vi "CreateFoldersRecursively.vi"(8 "error in (no error)":errorcluster caption="错误输入（无错误）", 9 "permissions":i16=493 caption="权限" format="%.0b", 10 "maximum path length":i32=252 caption="路径长度上限", 11 "directory":path caption="目录") -> (0 "error out":errorcluster caption="错误输出", 2 "directories created":path[](array[path]) caption="创建的目录", 3 "directory copy":path caption="目录副本")   [LabVIEW 2019, in "Logger.lvclass"]
uses:
  <userlib>/Logger/Logger.lvclass
panel:
  in  "Long Path Message":string="由于操作系统限制，该完整路径包含过多字符，LabVIEW将无法创建该文件夹。" caption="长路径信息"
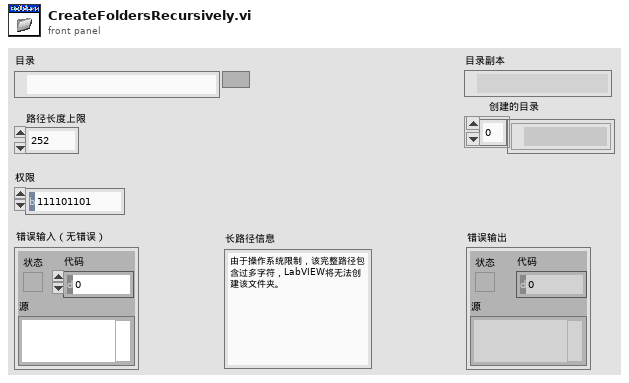
[diagram p1: front panel]
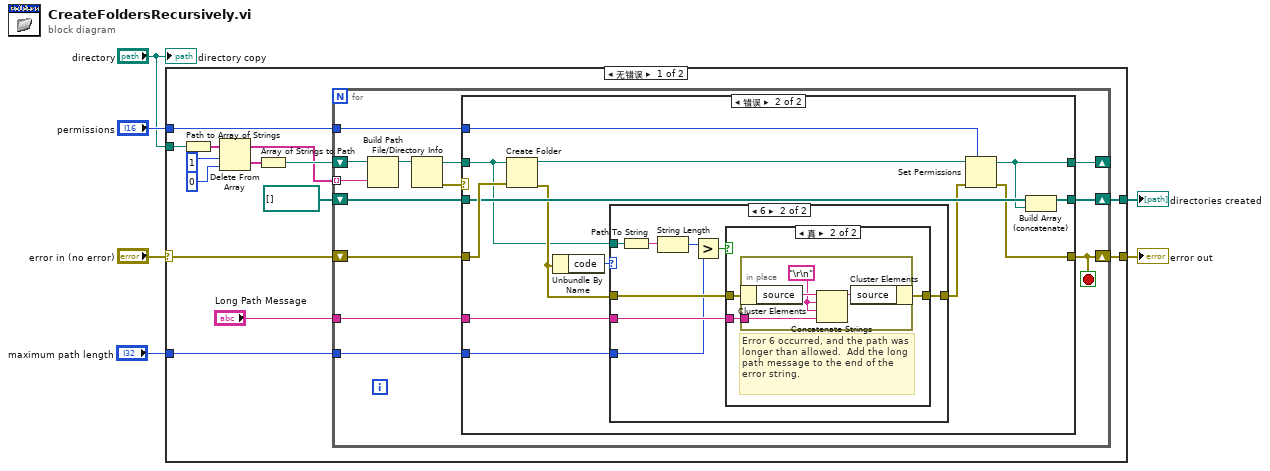
[diagram p0: block diagram]
diagram:
  n1 = case shown="无错误" "error in (no error)" {
    selector: "error in (no error)" -> [w9 w67]
    tunnel: [w20 w67] -> w6
    tunnel: "permissions" -> [w19 _]
    tunnel: [w15 _] -> w4
    tunnel: "directory" -> [w12 _]
    tunnel: "maximum path length" -> [w7 _]
    frame No Error {
      n2 = Path to Array of Strings(0:w12) -> (2:w18:string[])  [unwired: 1 out]
      n3 = Delete From Array(array=w18, length=1, index=0) -> (deleted portion=w13:string[], array with subset deleted=w10:string[])
      n4 = Array of Strings to Path(0:w13) -> (2:w17:path)  [unwired: 1 out]
      n5 = for {
        shift-right: [w29] -> _
        shift-left: w17 -> [w33]
        tunnel: w10 -> [w32] mode=indexing
        shift-right: [w23] -> w20
        shift-left: w9 -> [w28]
        tunnel: w19 -> [w27]
        shift-right: [w25] -> w15
        shift-left: path[] [] ("Array Constant") -> [w26]
        tunnel: "Long Path Message" -> [w22]
        tunnel: w7 -> [w21]
        stop <- w23 stop-if-true
        n6 = Build Path(base path=w33, name or relative path=w32) -> (appended path=w31:path)
        n7 = File/Directory Info(path=w31) -> (path out=w30:path, error out=w24:errorcluster)  [unwired: 1 in, 5 out]
        n8 = case shown="错误" w24 {
          tunnel: [w36 w43] -> w29
          tunnel: w30 -> [w36 w39]
          tunnel: w28 -> [w35 w49]
          tunnel: [w35 w44] -> w23
          tunnel: w27 -> [_ w48]
          tunnel: w26 -> [w34 w47]
          tunnel: [w34 w46] -> w25
          tunnel: w22 -> [_ w38]
          tunnel: w21 -> [_ w37]
          frame No Error {
          }
          frame Error {
            n9 = Create Folder(path (use dialog)=w39, error in=w49) -> (created path=w45:path, error out=w41:errorcluster)  [unwired: 2 out]
            n10 = Unbundle By Name(w41) -> ("code"=w42:i32)
            n11 = case shown="6" w42 {
              tunnel: w41 -> [w50 w56]
              tunnel: [w50 w55] -> w40
              tunnel: w39 -> [_ w58]
              tunnel: w38 -> [_ w54]
              tunnel: w37 -> [_ w51]
              frame Default {
              }
              frame 6 {
                n12 = Path To String(path=w58) -> (string=w57:string)
                n13 = String Length(string=w57) -> (length=w52:i32)
                n14 = Greater?(x=w52, y=w51) -> (0:w53:bool)
                n15 = case shown="真" w53 {
                  tunnel: w56 -> [w59 w62]
                  tunnel: [w59 w61] -> w55
                  tunnel: w54 -> [_ w60]
                  frame False {
                  }
                  frame True {
                    # "Error 6 occurred, and the path was longer than allowed.  Add the long path message to the end of the error string."
                    n16 = in-place {
                      in-place-border: w60 -> [w64]
                      w63 = "\r\n"
                      n17 = in-place-cluster #1(w62) -> ("source"=w66:string)
                      n18 = Concatenate Strings(w66, w63, w63, w64) -> (w65:string)
                      n19 = in-place-cluster #1("source"=w65) -> (w61:errorcluster)
                    }
                  }
                }
              }
            }
            n20 = Set Permissions(7:w48, 8:w40, 11:w45) -> (0:w44:errorcluster, 3:w43:path)  [unwired: 2 out]
            n21 = Build Array (concatenate)(w47, w43) -> (w46:path[])
          }
        }
      }
    }
    frame Error {
    }
  }
  "error out" <- w6
  "directories created" <- w4
  "directory copy" <- "directory"
